vi "Autonomous Independent.vi"() -> ()   [LabVIEW 2017]
doc: "This VI is called when autonomous begins, and will automatically be terminated when autonomous ends. You can carry out timed or sensor driven robot movement independently without needing to return to the caller."
uses:
  <vilib>/Rock Robotics/WPI/Utilities/WPI_GetSetVariantRefNum.vi
  <vilib>/Rock Robotics/Network Tables/NT Read String.vi
  <vilib>/Rock Robotics/WPI/RobotDrive/WPI_RobotDriveArcadeDrive_Standard(NoSaturation).vi
  <vilib>/Rock Robotics/Network Tables/NT Write Numeric Array.vi
  <vilib>/Rock Robotics/Network Tables/NT Read Number.vi
panel:
  out "Motor Values":dbl[](array[numeric])
  out "Current Movement, for debugging":T1 {"Y Joystick Value" scale=1.0..-1.0; "X Joystick Value" scale=-1.0..1.0}
  in  "Array of robot movements":T2(array[cluster])=[{"X Joystick Value"=0.39393939393939403, "Y Joystick Value"=0.0, "Delay (sec)"=1.0, "Movement Name"="turn"}, {"X Joystick Value"=-0.3737373737373737, "Y Joystick Value"=0.0, "Delay (sec)"=1.0, "Movement Name"="turn back"}] {"Y Joystick Value" scale=1.0..-1.0; "X Joystick Value" scale=-1.0..1.0}
  # "Be sure to right-click and choose Data Operations>>Make Current Value default if you want to save the array values with the VI"
  # "."
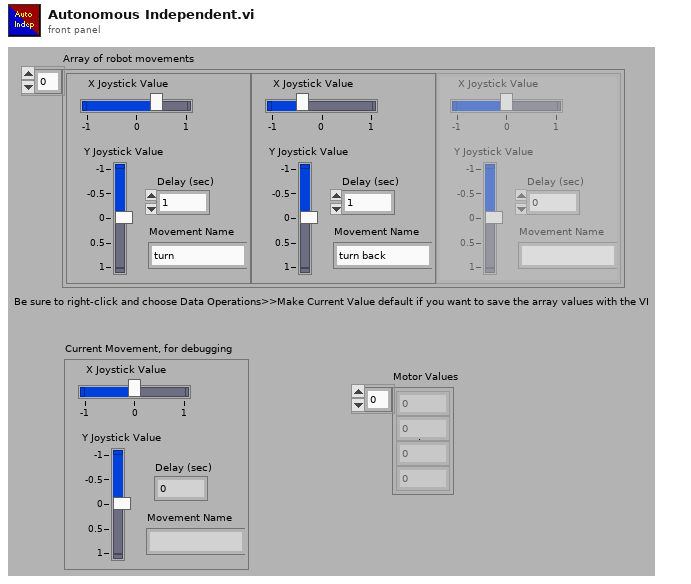
[diagram p1: front panel]
types:
  T1 = cluster{"X Joystick Value":dbl, "Y Joystick Value":dbl, "Delay (sec)":dbl, "Movement Name":string}
  T2 = cluster{"X Joystick Value":dbl, "Y Joystick Value":dbl, "Delay (sec)":dbl, "Movement Name":string}[]
  T3 = typedef "WPI_JoystickDevRef.ctl" = cluster{"Device":T4}
  T4 = typedef "WPI_JoystickDeviceEnum.ctl" = enum16{"USB 0", "USB 1", "USB 2", "USB 3", "USB 4", "USB 5"}
  T5 = typedef "WPI_RobotDriveDevRef.ctl" = cluster{"DevStatus":errorcluster, "Motors[]":T6[], "Square Inputs":bool, "Max Output":dbl}
  T6 = typedef "WPI_MotorControlDeviceRef.ctl" = cluster{"DeviceStatus":errorcluster, "Type":T7, "PWM":cluster{"PWM Channel":T8, "DeadBand":T9}, "CAN":cluster{"Device Number":u8, "SetOutput VI Ref":variant, "GetOutput VI Ref":variant, "Enable VI Ref":variant, "Disable VI Ref":variant, "Data":variant}, "Invert":bool, "DIO PWM":cluster{"PWM \"Enable\" Channel":T8, "DIOChannel":T10, "PWM Rate":dbl}}
  T7 = typedef "WPI_MotorControlType.ctl" = enum16{"PWM", "CAN", "DIO PWM"}
  T8 = typedef "FPGA_DIOPWMChannel.ctl" = enum8{"PWM 0", "PWM 1", "PWM 2", "PWM 3", "PWM 4", "PWM 5", "PWM 6", "PWM 7", "PWM 8", "PWM 9", "PWM MXP 0", "PWM MXP 1", "PWM MXP 2", "PWM MXP 3", "PWM MXP 4", "PWM MXP 5", "PWM MXP 6", "PWM MXP 7", "PWM MXP 8", "PWM MXP 9", "Invalid"}
  T9 = typedef "WPI_PWMDeadband.ctl" = cluster{"Name":string, "maxPositivePwm":i32, "minPositivePwm":i32, "centerPwm":i32, "maxNegativePwm":i32, "minNegativePwm":i32, "angularRange":u16}
  T10 = typedef "FPGA_DIOChannel.ctl" = enum8{"DIO 0", "DIO 1", "DIO 2", "DIO 3", "DIO 4", "DIO 5", "DIO 6", "DIO 7", "DIO 8", "DIO 9", "DIO MXP 0", "DIO MXP 1", "DIO MXP 2", "DIO MXP 3", "DIO MXP 4", "DIO MXP 5", "DIO MXP 6", "DIO MXP 7", "DIO MXP 8", "DIO MXP 9", "DIO MXP 10", "DIO MXP 11", "DIO MXP 12", "DIO MXP 13", "DIO MXP 14", "DIO MXP 15", "SPI Port CS1", "SPI Port CS2", "SPI Port CS3", "SPI Port MISO", "SPI Port MOSI", "Invalid"}
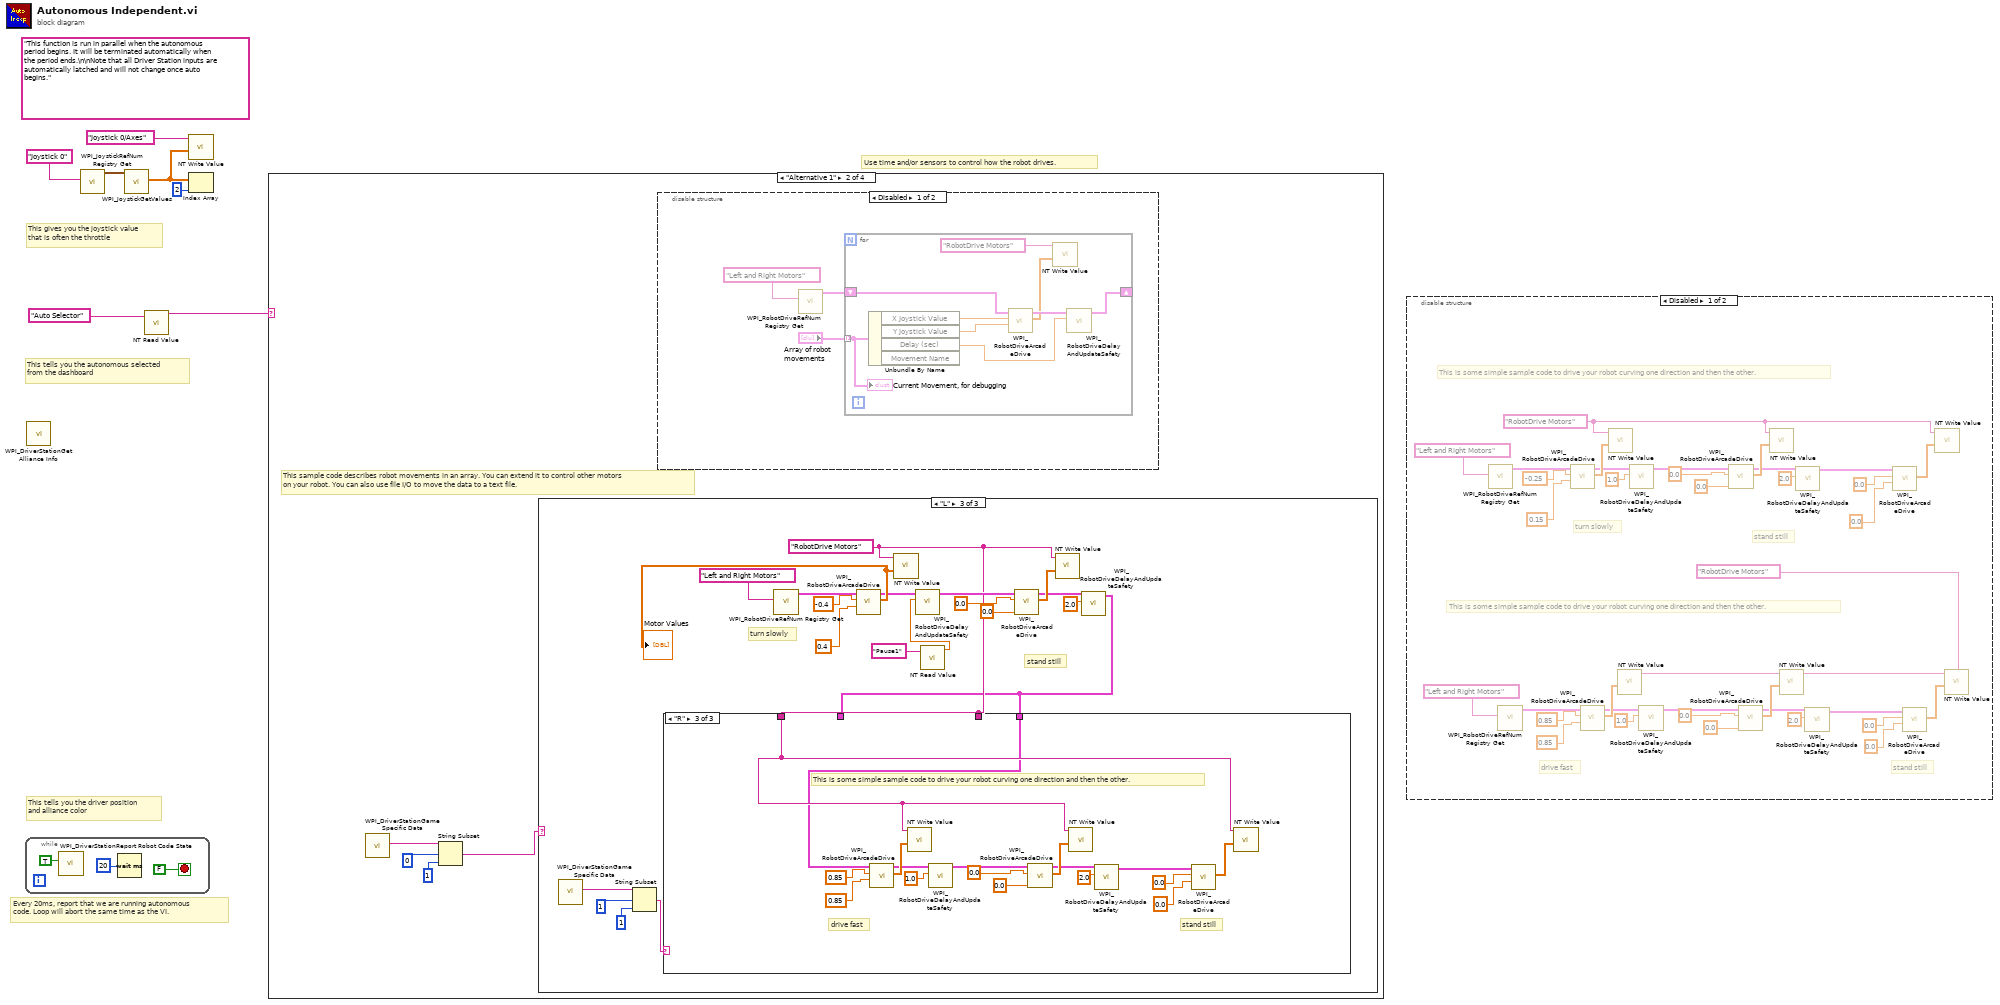
[diagram p0: block diagram]
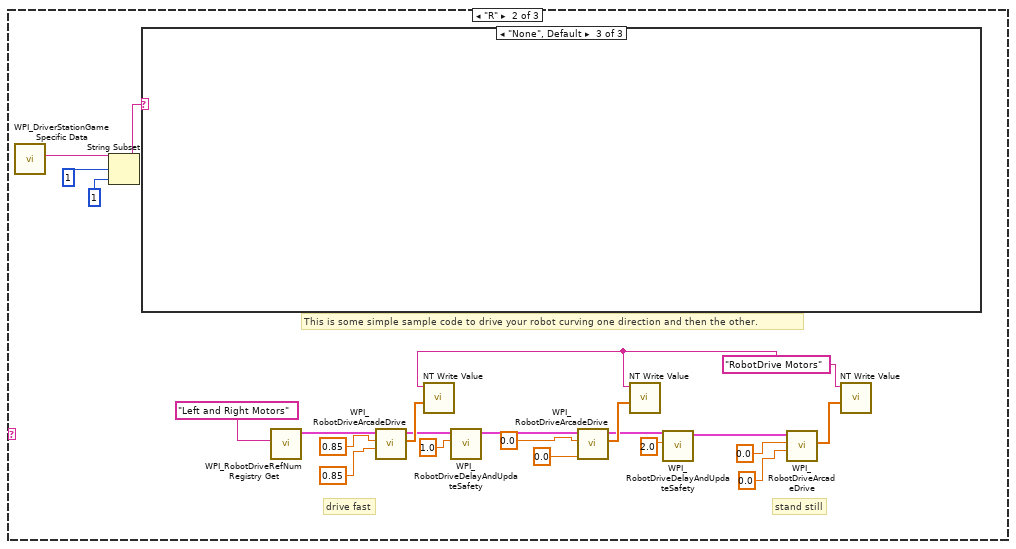
[diagram p6: hidden frame]
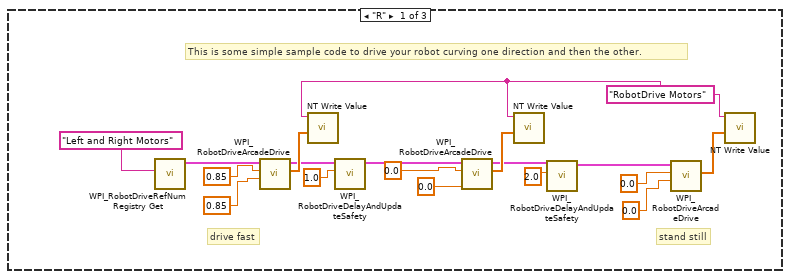
[diagram p7: hidden frame]
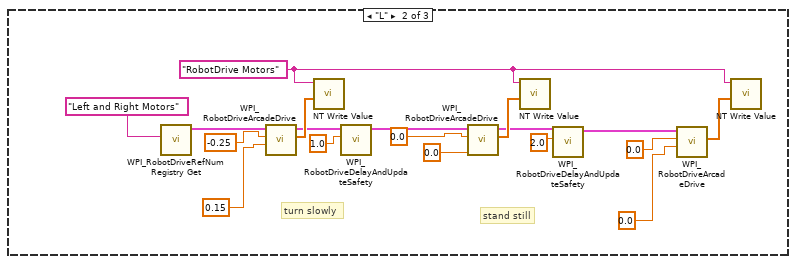
[diagram p8: hidden frame]
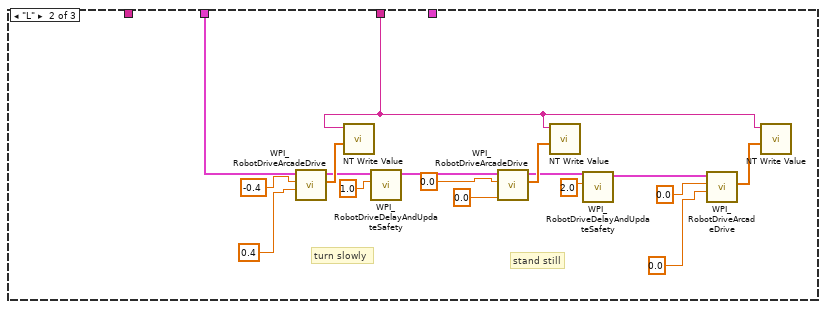
[diagram p10: hidden frame]
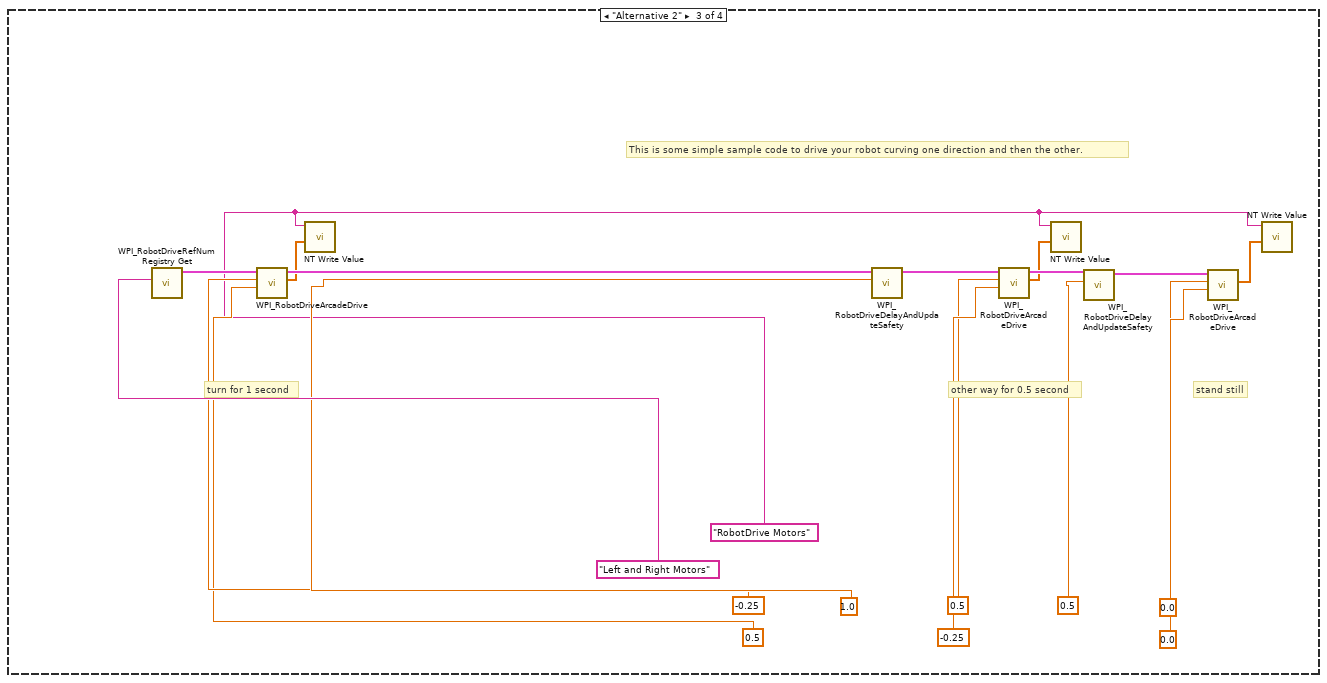
[diagram p11: hidden frame]
diagram:
  (unwired) "This function is run in parallel when the autonomous period begins. It will be terminated automatically when the period ends.\n\nNote that all Driver Station inputs are automatically latched and will not change once auto begins."
  # "This tells you the autonomous selected\nfrom the dashboard"
  # "Every 20ms, report that we are running autonomous\ncode. Loop will abort the same time as the VI."
  # "This gives you the joystick value\nthat is often the throttle"
  # "Use time and/or sensors to control how the robot drives."
  # "This tells you the driver position\nand alliance color"
  n1 = while {
    stop <- FALSE stop-if-true
    n2 = call <vilib>:"WPI_DriverStationReport Robot Code State.vi"("Autonomous"=TRUE) -> ()  [unwired: 10 in, 1 out]
    n3 = Wait (ms)(milliseconds to wait=u32 20) -> ()  [unwired: 1 out]
  }
  n4 = call <vilib>:"WPI_DriverStationGet Alliance Info.vi"() -> ()  [unwired: 12 out]
  n5 = call <vilib>:"WPI_JoystickRefNum Registry Get.vi"("refnum name"="Joystick 0") -> ("JoystickDevRef"=w6:T3)  [unwired: 1 in, 9 out]
  n6 = call <vilib>:"WPI_JoystickGetValues.vi"("JoystickDevRef"=w6) -> ("Axes"=w2:dbl[])  [unwired: 6 in, 4 out]
  n7 = call-poly <vilib>:"NT Read Value.vi"("Name"="Auto Selector") -> ("String"=w3:string)  [unwired: 9 in, 1 out]
  n8 = call-poly <vilib>:"NT Write Value.vi"("Numeric Array"=w2, "Name"="Joystick 0/Axes") -> ()  [unwired: 9 in, 1 out]
  n9 = Index Array(array=w2, index=2) -> ()  [unwired: 1 out]
  n10 = case shown="\"Alternative 1\"" w3 {
    frame Default {
      # "You can put your main auto here, or you can right-click on the case and make any\nother frame be the default case."
      # "This is the frame that will execute if no selection is made, or if it is not recognized"
    }
    frame "Alternative 1" {
      # "This sample code describes robot movements in an array. You can extend it to control other motors\non your robot. You can also use file I/O to move the data to a text file."
      n11 = call <vilib>:"WPI_DriverStationGame Specific Data.vi"() -> ("Game Specific Data"=w14:string)  [unwired: 11 in]
      n12 = String Subset(string=w14, offset (0)=0, length (rest)=1) -> (substring=w11:string)
      n13 = case shown="\"L\"" w11 {
        frame "None", Default {
        }
        frame "R" {
          w31 = "RobotDrive Motors" ("Name")
          # "This is some simple sample code to drive your robot curving one direction and then the other."
          # "stand still"
          # "drive fast"
          n14 = call <vilib>:"WPI_DriverStationGame Specific Data.vi"() -> ("Game Specific Data"=w30:string)  [unwired: 11 in]
          n15 = String Subset(string=w30, offset (0)=1, length (rest)=1) -> (substring=w27:string)
          n16 = case shown="\"None\", Default" w27 {
            frame "R" {
              w49 = "RobotDrive Motors" ("Name")
              # "This is some simple sample code to drive your robot curving one direction and then the other."
              # "stand still"
              # "drive fast"
              n17 = call <vilib>:"WPI_RobotDriveRefNum Registry Get.vi"("refnum name"="Left and Right Motors") -> ("RobotDriveDevRef"=w59:T5)  [unwired: 1 in, 9 out]
              n18 = call-poly <vilib>:"WPI_RobotDriveArcadeDrive.vi"("Y axis value"=0.85 ("X axis value"), "X axis value"=0.85, "RobotDriveDevRef"=w59) -> ("Motor Values"=w66:dbl[], "RobotDriveDevRef"=w63:T5)  [unwired: 1 in, 6 out]
              n19 = call-poly <vilib>:"NT Write Value.vi"("Numeric Array"=w66, "Name"=w49) -> ()  [unwired: 9 in, 1 out]
              n20 = call <vilib>:"WPI_RobotDriveDelayAndUpdateSafety.vi"("Delay (s)"=1.0, "RobotDriveDevRef"=w63) -> ("RobotDriveDevRef 2"=w62:T5)  [unwired: 8 in, 1 out]
              n21 = call-poly <vilib>:"WPI_RobotDriveArcadeDrive.vi"("Y axis value"=0.0 ("X axis value"), "X axis value"=0.0, "RobotDriveDevRef"=w62) -> ("Motor Values"=w65:dbl[], "RobotDriveDevRef"=w61:T5)  [unwired: 1 in, 6 out]
              n22 = call-poly <vilib>:"NT Write Value.vi"("Numeric Array"=w65, "Name"=w49) -> ()  [unwired: 9 in, 1 out]
              n23 = call <vilib>:"WPI_RobotDriveDelayAndUpdateSafety.vi"("Delay (s)"=2.0, "RobotDriveDevRef"=w61) -> ("RobotDriveDevRef 2"=w60:T5)  [unwired: 8 in, 1 out]
              n24 = call-poly <vilib>:"WPI_RobotDriveArcadeDrive.vi"("Y axis value"=0.0 ("X axis value"), "X axis value"=0.0, "RobotDriveDevRef"=w60) -> ("Motor Values"=w64:dbl[])  [unwired: 1 in, 7 out]
              n25 = call-poly <vilib>:"NT Write Value.vi"("Numeric Array"=w64, "Name"=w49) -> ()  [unwired: 9 in, 1 out]
            }
            frame "L" {
              w68 = "RobotDrive Motors" ("Name")
              # "stand still"
              # "turn slowly"
              n26 = call <vilib>:"WPI_RobotDriveRefNum Registry Get.vi"("refnum name"="Left and Right Motors") -> ("RobotDriveDevRef"=w77:T5)  [unwired: 1 in, 9 out]
              n27 = call-poly <vilib>:"WPI_RobotDriveArcadeDrive.vi"("Y axis value"=0.15 ("X axis value"), "X axis value"=-0.25, "RobotDriveDevRef"=w77) -> ("Motor Values"=w84:dbl[], "RobotDriveDevRef"=w81:T5)  [unwired: 1 in, 6 out]
              n28 = call-poly <vilib>:"NT Write Value.vi"("Numeric Array"=w84, "Name"=w68) -> ()  [unwired: 9 in, 1 out]
              n29 = call <vilib>:"WPI_RobotDriveDelayAndUpdateSafety.vi"("Delay (s)"=1.0, "RobotDriveDevRef"=w81) -> ("RobotDriveDevRef 2"=w80:T5)  [unwired: 8 in, 1 out]
              n30 = call-poly <vilib>:"WPI_RobotDriveArcadeDrive.vi"("Y axis value"=0.0 ("X axis value"), "X axis value"=0.0, "RobotDriveDevRef"=w80) -> ("Motor Values"=w83:dbl[], "RobotDriveDevRef"=w79:T5)  [unwired: 1 in, 6 out]
              n31 = call-poly <vilib>:"NT Write Value.vi"("Numeric Array"=w83, "Name"=w68) -> ()  [unwired: 9 in, 1 out]
              n32 = call <vilib>:"WPI_RobotDriveDelayAndUpdateSafety.vi"("Delay (s)"=2.0, "RobotDriveDevRef"=w79) -> ("RobotDriveDevRef 2"=w78:T5)  [unwired: 8 in, 1 out]
              n33 = call-poly <vilib>:"WPI_RobotDriveArcadeDrive.vi"("Y axis value"=0.0 ("X axis value"), "X axis value"=0.0, "RobotDriveDevRef"=w78) -> ("Motor Values"=w82:dbl[])  [unwired: 1 in, 7 out]
              n34 = call-poly <vilib>:"NT Write Value.vi"("Numeric Array"=w82, "Name"=w68) -> ()  [unwired: 9 in, 1 out]
            }
            frame "None", Default {
            }
          }
          n35 = call <vilib>:"WPI_RobotDriveRefNum Registry Get.vi"("refnum name"="Left and Right Motors") -> ("RobotDriveDevRef"=w41:T5)  [unwired: 1 in, 9 out]
          n36 = call-poly <vilib>:"WPI_RobotDriveArcadeDrive.vi"("Y axis value"=0.85 ("X axis value"), "X axis value"=0.85, "RobotDriveDevRef"=w41) -> ("Motor Values"=w48:dbl[], "RobotDriveDevRef"=w45:T5)  [unwired: 1 in, 6 out]
          n37 = call-poly <vilib>:"NT Write Value.vi"("Numeric Array"=w48, "Name"=w31) -> ()  [unwired: 9 in, 1 out]
          n38 = call <vilib>:"WPI_RobotDriveDelayAndUpdateSafety.vi"("Delay (s)"=1.0, "RobotDriveDevRef"=w45) -> ("RobotDriveDevRef 2"=w44:T5)  [unwired: 8 in, 1 out]
          n39 = call-poly <vilib>:"WPI_RobotDriveArcadeDrive.vi"("Y axis value"=0.0 ("X axis value"), "X axis value"=0.0, "RobotDriveDevRef"=w44) -> ("Motor Values"=w47:dbl[], "RobotDriveDevRef"=w43:T5)  [unwired: 1 in, 6 out]
          n40 = call-poly <vilib>:"NT Write Value.vi"("Numeric Array"=w47, "Name"=w31) -> ()  [unwired: 9 in, 1 out]
          n41 = call <vilib>:"WPI_RobotDriveDelayAndUpdateSafety.vi"("Delay (s)"=2.0, "RobotDriveDevRef"=w43) -> ("RobotDriveDevRef 2"=w42:T5)  [unwired: 8 in, 1 out]
          n42 = call-poly <vilib>:"WPI_RobotDriveArcadeDrive.vi"("Y axis value"=0.0 ("X axis value"), "X axis value"=0.0, "RobotDriveDevRef"=w42) -> ("Motor Values"=w46:dbl[])  [unwired: 1 in, 7 out]
          n43 = call-poly <vilib>:"NT Write Value.vi"("Numeric Array"=w46, "Name"=w31) -> ()  [unwired: 9 in, 1 out]
        }
        frame "L" {
          w88 = "RobotDrive Motors" ("Name")
          # "stand still"
          # "turn slowly"
          n44 = call <vilib>:"WPI_DriverStationGame Specific Data.vi"() -> ("Game Specific Data"=w92:string)  [unwired: 11 in]
          n45 = String Subset(string=w92, offset (0)=1, length (rest)=1) -> (substring=w89:string)
          n46 = call <vilib>:"WPI_RobotDriveRefNum Registry Get.vi"("refnum name"="Left and Right Motors") -> ("RobotDriveDevRef"=w99:T5)  [unwired: 1 in, 9 out]
          n47 = call-poly <vilib>:"WPI_RobotDriveArcadeDrive.vi"("Y axis value"=0.4 ("X axis value"), "X axis value"=-0.4, "RobotDriveDevRef"=w99) -> ("Motor Values"=w104:dbl[], "RobotDriveDevRef"=w102:T5)  [unwired: 1 in, 6 out]
          "Motor Values" <- w104
          n48 = call-poly <vilib>:"NT Write Value.vi"("Numeric Array"=w104, "Name"=w88) -> ()  [unwired: 9 in, 1 out]
          n49 = call-poly <vilib>:"NT Read Value.vi"("Name"="Pause1") -> ("Numeric"=w85:dbl)  [unwired: 9 in, 1 out]
          n50 = call <vilib>:"WPI_RobotDriveDelayAndUpdateSafety.vi"("Delay (s)"=w85, "RobotDriveDevRef"=w102) -> ("RobotDriveDevRef 2"=w101:T5)  [unwired: 8 in, 1 out]
          n51 = call-poly <vilib>:"WPI_RobotDriveArcadeDrive.vi"("Y axis value"=0.0 ("X axis value"), "X axis value"=0.0, "RobotDriveDevRef"=w101) -> ("Motor Values"=w103:dbl[], "RobotDriveDevRef"=w100:T5)  [unwired: 1 in, 6 out]
          n52 = call-poly <vilib>:"NT Write Value.vi"("Numeric Array"=w103, "Name"=w88) -> ()  [unwired: 9 in, 1 out]
          n53 = call <vilib>:"WPI_RobotDriveDelayAndUpdateSafety.vi"("Delay (s)"=2.0, "RobotDriveDevRef"=w100) -> ("RobotDriveDevRef 2"=w87:T5)  [unwired: 8 in, 1 out]
          n54 = case shown="\"R\"" w89 {
            tunnel: w87 -> [_ w106 _]
            tunnel: w88 -> [_ w105 _]
            tunnel: w88 -> [_ _ w123]
            tunnel: w87 -> [_ _ w122]
            frame "None", Default {
            }
            frame "L" {
              # "stand still"
              # "turn slowly"
              n55 = call-poly <vilib>:"WPI_RobotDriveArcadeDrive.vi"("Y axis value"=0.4 ("X axis value"), "X axis value"=-0.4, "RobotDriveDevRef"=w106) -> ("Motor Values"=w121:dbl[], "RobotDriveDevRef"=w118:T5)  [unwired: 1 in, 6 out]
              n56 = call-poly <vilib>:"NT Write Value.vi"("Numeric Array"=w121, "Name"=w105) -> ()  [unwired: 9 in, 1 out]
              n57 = call <vilib>:"WPI_RobotDriveDelayAndUpdateSafety.vi"("Delay (s)"=1.0, "RobotDriveDevRef"=w118) -> ("RobotDriveDevRef 2"=w107:T5)  [unwired: 8 in, 1 out]
              n58 = call-poly <vilib>:"WPI_RobotDriveArcadeDrive.vi"("Y axis value"=0.0 ("X axis value"), "X axis value"=0.0, "RobotDriveDevRef"=w107) -> ("Motor Values"=w120:dbl[], "RobotDriveDevRef"=w117:T5)  [unwired: 1 in, 6 out]
              n59 = call-poly <vilib>:"NT Write Value.vi"("Numeric Array"=w120, "Name"=w105) -> ()  [unwired: 9 in, 1 out]
              n60 = call <vilib>:"WPI_RobotDriveDelayAndUpdateSafety.vi"("Delay (s)"=2.0, "RobotDriveDevRef"=w117) -> ("RobotDriveDevRef 2"=w116:T5)  [unwired: 8 in, 1 out]
              n61 = call-poly <vilib>:"WPI_RobotDriveArcadeDrive.vi"("Y axis value"=0.0 ("X axis value"), "X axis value"=0.0, "RobotDriveDevRef"=w116) -> ("Motor Values"=w119:dbl[])  [unwired: 1 in, 7 out]
              n62 = call-poly <vilib>:"NT Write Value.vi"("Numeric Array"=w119, "Name"=w105) -> ()  [unwired: 9 in, 1 out]
            }
            frame "R" {
              # "This is some simple sample code to drive your robot curving one direction and then the other."
              # "stand still"
              # "drive fast"
              n63 = call-poly <vilib>:"WPI_RobotDriveArcadeDrive.vi"("Y axis value"=0.85 ("X axis value"), "X axis value"=0.85, "RobotDriveDevRef"=w122) -> ("Motor Values"=w138:dbl[], "RobotDriveDevRef"=w135:T5)  [unwired: 1 in, 6 out]
              n64 = call-poly <vilib>:"NT Write Value.vi"("Numeric Array"=w138, "Name"=w123) -> ()  [unwired: 9 in, 1 out]
              n65 = call <vilib>:"WPI_RobotDriveDelayAndUpdateSafety.vi"("Delay (s)"=1.0, "RobotDriveDevRef"=w135) -> ("RobotDriveDevRef 2"=w134:T5)  [unwired: 8 in, 1 out]
              n66 = call-poly <vilib>:"WPI_RobotDriveArcadeDrive.vi"("Y axis value"=0.0 ("X axis value"), "X axis value"=0.0, "RobotDriveDevRef"=w134) -> ("Motor Values"=w137:dbl[], "RobotDriveDevRef"=w133:T5)  [unwired: 1 in, 6 out]
              n67 = call-poly <vilib>:"NT Write Value.vi"("Numeric Array"=w137, "Name"=w123) -> ()  [unwired: 9 in, 1 out]
              n68 = call <vilib>:"WPI_RobotDriveDelayAndUpdateSafety.vi"("Delay (s)"=2.0, "RobotDriveDevRef"=w133) -> ("RobotDriveDevRef 2"=w132:T5)  [unwired: 8 in, 1 out]
              n69 = call-poly <vilib>:"WPI_RobotDriveArcadeDrive.vi"("Y axis value"=0.0 ("X axis value"), "X axis value"=0.0, "RobotDriveDevRef"=w132) -> ("Motor Values"=w136:dbl[])  [unwired: 1 in, 7 out]
              n70 = call-poly <vilib>:"NT Write Value.vi"("Numeric Array"=w136, "Name"=w123) -> ()  [unwired: 9 in, 1 out]
            }
          }
        }
      }
      n71 = disable-structure shown="Disabled" {
        frame Disabled {
          n72 = call <vilib>:"WPI_RobotDriveRefNum Registry Get.vi"("refnum name"="Left and Right Motors") -> ("RobotDriveDevRef"=w16:T5)  [unwired: 1 in, 9 out]
          n73 = for {
            shift-right: [w24] -> _
            shift-left: w16 -> [w25]
            tunnel: "Array of robot movements" -> [w20] mode=indexing
            n74 = Unbundle By Name(w20) -> ("X Joystick Value"=w23:dbl, "Y Joystick Value"=w22:dbl, "Delay (sec)"=w21:dbl)  [unwired: 1 out]
            n75 = call-poly <vilib>:"WPI_RobotDriveArcadeDrive.vi"("Y axis value"=w22, "X axis value"=w23, "RobotDriveDevRef"=w25) -> ("Motor Values"=w18:dbl[], "RobotDriveDevRef"=w26:T5)  [unwired: 1 in, 6 out]
            n76 = call-poly <vilib>:"NT Write Value.vi"("Numeric Array"=w18, "Name"="RobotDrive Motors") -> ()  [unwired: 9 in, 1 out]
            n77 = call <vilib>:"WPI_RobotDriveDelayAndUpdateSafety.vi"("Delay (s)"=w21, "RobotDriveDevRef"=w26) -> ("RobotDriveDevRef 2"=w24:T5)  [unwired: 8 in, 1 out]
            "Current Movement, for debugging" <- w20
          }
        }
        frame Enabled {
        }
      }
    }
    frame "Alternative 2" {
      w140 = "RobotDrive Motors" ("Name")
      # "This is some simple sample code to drive your robot curving one direction and then the other."
      # "stand still"
      # "other way for 0.5 second"
      # "turn for 1 second"
      n78 = call <vilib>:"WPI_RobotDriveRefNum Registry Get.vi"("refnum name"="Left and Right Motors") -> ("RobotDriveDevRef"=w156:T5)  [unwired: 1 in, 9 out]
      n79 = call-poly <vilib>:"WPI_RobotDriveArcadeDrive.vi"("Y axis value"=0.5 ("X axis value"), "X axis value"=-0.25, "RobotDriveDevRef"=w156) -> ("Motor Values"=w139:dbl[], "RobotDriveDevRef"=w149:T5)  [unwired: 1 in, 6 out]
      n80 = call-poly <vilib>:"NT Write Value.vi"("Numeric Array"=w139, "Name"=w140) -> ()  [unwired: 9 in, 1 out]
      n81 = call <vilib>:"WPI_RobotDriveDelayAndUpdateSafety.vi"("Delay (s)"=1.0, "RobotDriveDevRef"=w149) -> ("RobotDriveDevRef 2"=w150:T5)  [unwired: 8 in, 1 out]
      n82 = call-poly <vilib>:"WPI_RobotDriveArcadeDrive.vi"("Y axis value"=-0.25 ("X axis value"), "X axis value"=0.5, "RobotDriveDevRef"=w150) -> ("Motor Values"=w141:dbl[], "RobotDriveDevRef"=w151:T5)  [unwired: 1 in, 6 out]
      n83 = call-poly <vilib>:"NT Write Value.vi"("Numeric Array"=w141, "Name"=w140) -> ()  [unwired: 9 in, 1 out]
      n84 = call <vilib>:"WPI_RobotDriveDelayAndUpdateSafety.vi"("Delay (s)"=0.5, "RobotDriveDevRef"=w151) -> ("RobotDriveDevRef 2"=w152:T5)  [unwired: 8 in, 1 out]
      n85 = call-poly <vilib>:"WPI_RobotDriveArcadeDrive.vi"("Y axis value"=0.0 ("X axis value"), "X axis value"=0.0, "RobotDriveDevRef"=w152) -> ("Motor Values"=w142:dbl[])  [unwired: 1 in, 7 out]
      n86 = call-poly <vilib>:"NT Write Value.vi"("Numeric Array"=w142, "Name"=w140) -> ()  [unwired: 9 in, 1 out]
    }
    frame "Your Turn" {
    }
  }
  n87 = disable-structure shown="Disabled" {
    frame Disabled {
      w158 = "RobotDrive Motors" ("Name")
      w176 = "RobotDrive Motors" ("Name")
      # "This is some simple sample code to drive your robot curving one direction and then the other."
      # "stand still"
      # "drive fast"
      # "This is some simple sample code to drive your robot curving one direction and then the other."
      # "stand still"
      # "turn slowly"
      n88 = call <vilib>:"WPI_RobotDriveRefNum Registry Get.vi"("refnum name"="Left and Right Motors") -> ("RobotDriveDevRef"=w185:T5)  [unwired: 1 in, 9 out]
      n89 = call <vilib>:"WPI_RobotDriveRefNum Registry Get.vi"("refnum name"="Left and Right Motors") -> ("RobotDriveDevRef"=w168:T5)  [unwired: 1 in, 9 out]
      n90 = call-poly <vilib>:"WPI_RobotDriveArcadeDrive.vi"("Y axis value"=0.15 ("X axis value"), "X axis value"=-0.25, "RobotDriveDevRef"=w185) -> ("Motor Values"=w192:dbl[], "RobotDriveDevRef"=w189:T5)  [unwired: 1 in, 6 out]
      n91 = call-poly <vilib>:"WPI_RobotDriveArcadeDrive.vi"("Y axis value"=0.85 ("X axis value"), "X axis value"=0.85, "RobotDriveDevRef"=w168) -> ("Motor Values"=w175:dbl[], "RobotDriveDevRef"=w172:T5)  [unwired: 1 in, 6 out]
      n92 = call-poly <vilib>:"NT Write Value.vi"("Numeric Array"=w192, "Name"=w176) -> ()  [unwired: 9 in, 1 out]
      n93 = call-poly <vilib>:"NT Write Value.vi"("Numeric Array"=w175, "Name"=w158) -> ()  [unwired: 9 in, 1 out]
      n94 = call <vilib>:"WPI_RobotDriveDelayAndUpdateSafety.vi"("Delay (s)"=1.0, "RobotDriveDevRef"=w189) -> ("RobotDriveDevRef 2"=w188:T5)  [unwired: 8 in, 1 out]
      n95 = call <vilib>:"WPI_RobotDriveDelayAndUpdateSafety.vi"("Delay (s)"=1.0, "RobotDriveDevRef"=w172) -> ("RobotDriveDevRef 2"=w171:T5)  [unwired: 8 in, 1 out]
      n96 = call-poly <vilib>:"WPI_RobotDriveArcadeDrive.vi"("Y axis value"=0.0 ("X axis value"), "X axis value"=0.0, "RobotDriveDevRef"=w188) -> ("Motor Values"=w191:dbl[], "RobotDriveDevRef"=w187:T5)  [unwired: 1 in, 6 out]
      n97 = call-poly <vilib>:"WPI_RobotDriveArcadeDrive.vi"("Y axis value"=0.0 ("X axis value"), "X axis value"=0.0, "RobotDriveDevRef"=w171) -> ("Motor Values"=w174:dbl[], "RobotDriveDevRef"=w170:T5)  [unwired: 1 in, 6 out]
      n98 = call-poly <vilib>:"NT Write Value.vi"("Numeric Array"=w191, "Name"=w176) -> ()  [unwired: 9 in, 1 out]
      n99 = call-poly <vilib>:"NT Write Value.vi"("Numeric Array"=w174, "Name"=w158) -> ()  [unwired: 9 in, 1 out]
      n100 = call <vilib>:"WPI_RobotDriveDelayAndUpdateSafety.vi"("Delay (s)"=2.0, "RobotDriveDevRef"=w187) -> ("RobotDriveDevRef 2"=w186:T5)  [unwired: 8 in, 1 out]
      n101 = call <vilib>:"WPI_RobotDriveDelayAndUpdateSafety.vi"("Delay (s)"=2.0, "RobotDriveDevRef"=w170) -> ("RobotDriveDevRef 2"=w169:T5)  [unwired: 8 in, 1 out]
      n102 = call-poly <vilib>:"WPI_RobotDriveArcadeDrive.vi"("Y axis value"=0.0 ("X axis value"), "X axis value"=0.0, "RobotDriveDevRef"=w186) -> ("Motor Values"=w190:dbl[])  [unwired: 1 in, 7 out]
      n103 = call-poly <vilib>:"WPI_RobotDriveArcadeDrive.vi"("Y axis value"=0.0 ("X axis value"), "X axis value"=0.0, "RobotDriveDevRef"=w169) -> ("Motor Values"=w173:dbl[])  [unwired: 1 in, 7 out]
      n104 = call-poly <vilib>:"NT Write Value.vi"("Numeric Array"=w190, "Name"=w176) -> ()  [unwired: 9 in, 1 out]
      n105 = call-poly <vilib>:"NT Write Value.vi"("Numeric Array"=w173, "Name"=w158) -> ()  [unwired: 9 in, 1 out]
    }
    frame Enabled {
    }
  }
